vi "ReadWrite.vi"(10 "Torque Write":dbl, 11 "Selector FGV":enum16{"Leer", "Escribir"}(ring)) -> (3 "Torque Read":dbl)   [LabVIEW 2020]
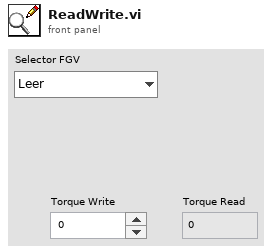
[diagram p1: front panel]
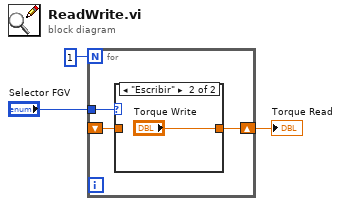
[diagram p0: block diagram]
diagram:
  n1 = for {
    N: 1 -> [_]
    shift-right: [w5] -> w1
    shift-left: _ -> [w4]
    tunnel: "Selector FGV" -> [w6]
    n2 = case shown="\"Escribir\"" w6 {
      tunnel: [w7 "Torque Write"] -> w5
      tunnel: w4 -> [w7 _]
      frame "Leer", Default {
      }
      frame "Escribir" {
      }
    }
  }
  "Torque Read" <- w1
